vi "RampTestwithPlateau.vi"() -> ()   [LabVIEW 2016]
panel:
  in  "Plateau time (ms)":dbl=1.0
  out "Step seperation (us)":dbl=8.0
  in  "Ramp duration (us)":dbl=400.0 format="%#_6f"
  in  "Ramp trigger source":T1(ring)=enum."BNC_IN_A_RISING"
  in  "Step Size (Hz)":dbl=10000.0 format="%#_6f"
  in  "End Frequency (Hz)":dbl=700000.0 format="%#_13g"
  in  "Starting Frequency (Hz)":dbl=200000.0 format="%#_6f"
  in  "Channels":T2(ring)=enum."Channel 1"
  out "return count":u32=368
  out "error out":errorcluster={"status"=TRUE, "code"=-1073807339, "source"="VISA Read in RampTest.vi"}
  out "read buffer":string="DDS reset OK (0, 0)\r\n"
  out "Final instruction string":string="dds 1 reset\rdcp 1 spi:CFR2=0x1000080\rdcp 1 spi:STP0=0xD1B71\rdcp 1 wait:0h:\rdcp 1 update:u\rdcp 1 spi:DRL=0x2DE00D000D1B71\rdcp 1 spi:DRSS=0xA7C60000A7C6\rdcp 1 spi:DRR=0x7D007D0\rdcp 1 spi:CFR2=0x80080\rdcp 1 wait::BNC_IN_A_RISING\rdcp 1 update:u+d\rdcp 1 wait:50000h:\rdcp 1 update:u\rdcp 1 spi:CFR2=0x1000080\rdcp 1 spi:STP0=0x2DE00D\rdcp 1 wait:0h:\rdcp 1 update:u\rdcp 1 start\r"
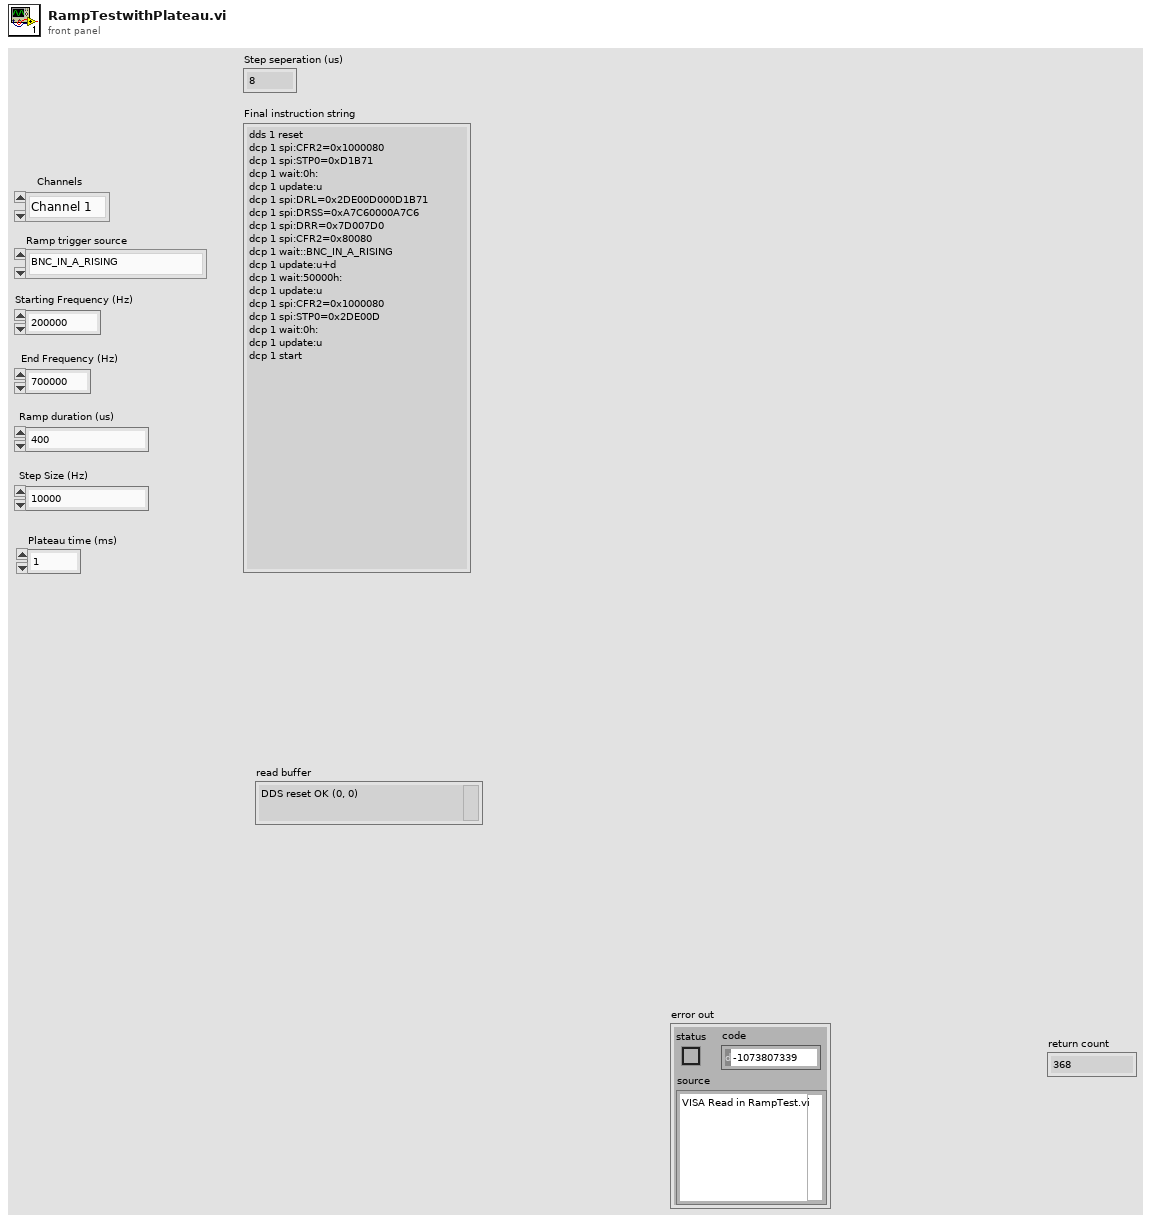
[diagram p1: front panel]
types:
  T1 = enum32{"O_RAMP_SWP_OVR", "RAM_SWP_OVR", "O_DROVER", "DROVER", "O_SPI_FIFO_EV1", "SPI_FIFO_EV1", "O_SPI_FIFO_EV0", "SPI_FIFO_EV0", "O_SPI_FIFO_FLUSHED", "SPI_FIFO_FLUSHED", "BNC_IN_B_LEVEL", "BNC_IN_B_FALLING", "BNC_IN_B_RISING", "BNC_IN_A_LEVEL", "BNC_IN_A_FALLING", "BNC_IN_A_RISING", "ALL_SPI_FIFOS_FLUSHED", "NONE"}
  T2 = enum32{"Channel 0", "Channel 1", "Both channels"}
  T3 = cluster{"Enable ASF from STP (F)":bool, "Digital ramp enable (F)":bool, "Digital ramp no-dwell high (F)":bool, "Digital ramp no-dwell low (F)":bool, "Matched latency enable (T)":bool, "Parallel data port enable (F)":bool}
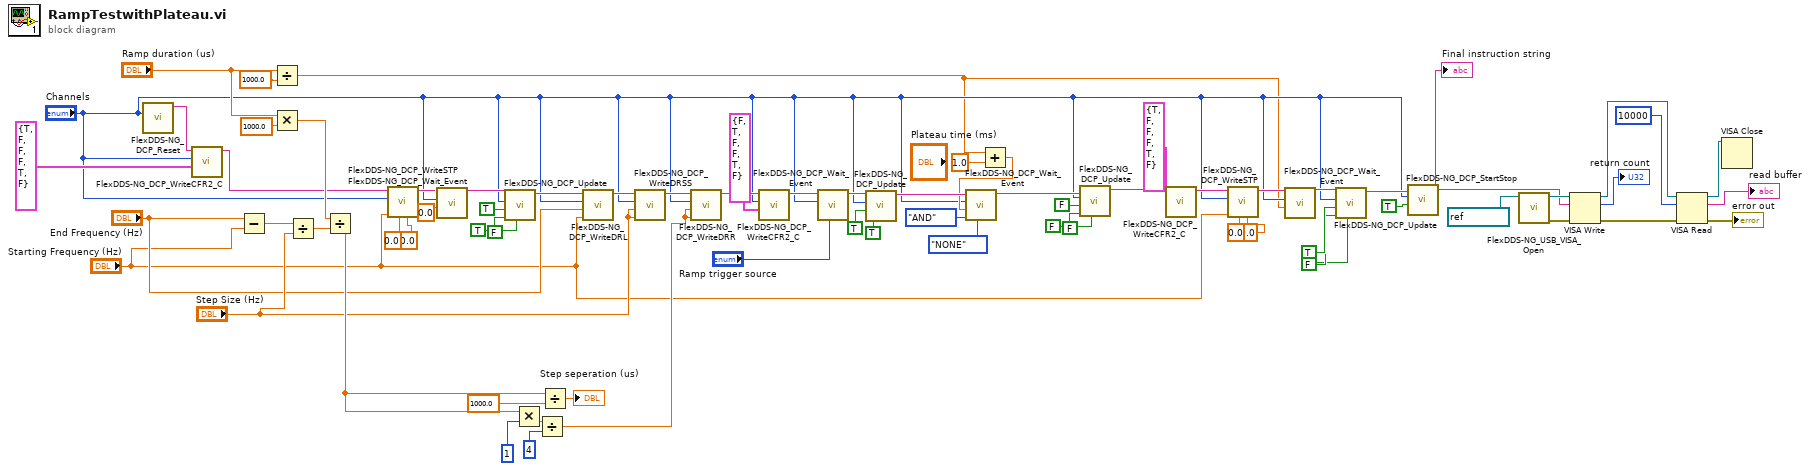
[diagram p0: block diagram]
diagram:
  n1 = call "FlexDDS-NG_DCP_Reset.vi"("Channels"="Channels") -> ("appended instruction string"=w22:string)  [unwired: 10 in]
  n2 = call "FlexDDS-NG_DCP_WriteCFR2_C.vi"("CFR2 bits"=T3 {"Enable ASF from STP (F)"=TRUE, "Digital ramp enable (F)"=FALSE, "Digital ramp no-dwell high (F)"=FALSE, "Digital ramp no-dwell low (F)"=FALSE, "Matched latency enable (T)"=TRUE, "Parallel data port enable (F)"=FALSE} ("CFR2 bits 2"), "Channels"="Channels", "initial instruction string"=w22) -> ("appended instruction string"=w23:string)  [unwired: 8 in]
  n3 = Subtract(x="End Frequency (Hz)", y="Starting Frequency (Hz)") -> (x-y=w35:dbl)
  n4 = Divide(x="Ramp duration (us)", y=1000.0) -> (x/y=w1:dbl)
  n5 = Multiply(x="Ramp duration (us)", y=1000.0) -> (x*y=w32:dbl)
  n6 = Divide(x=w35, y="Step Size (Hz)") -> (x/y=w33:dbl)
  n7 = Divide(x=w32, y=w33) -> (x/y=w31:dbl)
  n8 = call "FlexDDS-NG_DCP_WriteSTP.vi"("phase degrees (0..360)"=0.0, "amplitude (0..1)"=0.0, "frequency Hz (0..400M)"="Starting Frequency (Hz)", "Channels"="Channels", "initial instruction string"=w23) -> ("appended instruction string"=w16:string)  [unwired: 6 in]
  n9 = call "FlexDDS-NG_DCP_Wait_Event.vi"("waiting time [ms]"=0.0, "Channels in"="Channels", "appended instruction string in"=w16) -> ("appended instruction string"=w17:string)  [unwired: 8 in]
  n10 = call "FlexDDS-NG_DCP_Update.vi"("ONLY IO_UPDATE"=TRUE, "DRCTL(true=+, false=-)"=FALSE ("DRCTL(true=+, false=-) 2"), "IO_UPDATE(true=u, false = '')"=TRUE ("IO_UPDATE(true=u, false = '')  2"), "Channels"="Channels", "appended instruction string in"=w17) -> ("appended instruction string out"=w15:string)  [unwired: 6 in]
  n11 = Multiply(x=w31, y=u16 1) -> (x*y=w37:dbl)
  n12 = Divide(x=w37, y=u16 4) -> (x/y=w9:dbl)
  n13 = Divide(x=w31, y=1000.0 ("x/y")) -> (x/y=→"Step seperation (us)":dbl)
  n14 = call "FlexDDS-NG_DCP_WriteDRL.vi"("low limit"="Starting Frequency (Hz)", "high limit"="End Frequency (Hz)", "Channels"="Channels", "initial instruction string"=w15) -> ("appended instruction string"=w61:string)  [unwired: 7 in]
  n15 = call "FlexDDS-NG_DCP_WriteDRSS.vi"("increment step size"="Step Size (Hz)", "decrement step size"="Step Size (Hz)", "Channels"="Channels", "initial instruction string"=w61) -> ("appended instruction string"=w60:string)  [unwired: 7 in]
  n16 = call "FlexDDS-NG_DCP_WriteDRR.vi"("digital ramp positive slope rate"=w9, "digital ramp negative slope rate"=w9, "Channels"="Channels", "initial instruction string"=w60) -> ("appended instruction string"=w59:string)  [unwired: 7 in]
  n17 = call "FlexDDS-NG_DCP_WriteCFR2_C.vi"("CFR2 bits"=T3 {"Enable ASF from STP (F)"=FALSE, "Digital ramp enable (F)"=TRUE, "Digital ramp no-dwell high (F)"=FALSE, "Digital ramp no-dwell low (F)"=FALSE, "Matched latency enable (T)"=TRUE, "Parallel data port enable (F)"=FALSE}, "Channels"="Channels", "initial instruction string"=w59) -> ("appended instruction string"=w54:string)  [unwired: 8 in]
  n18 = call "FlexDDS-NG_DCP_Wait_Event.vi"("Event 1"="Ramp trigger source", "Channels in"="Channels", "appended instruction string in"=w54) -> ("appended instruction string"=w53:string)  [unwired: 8 in]
  n19 = call "FlexDDS-NG_DCP_Update.vi"("DRCTL(true=+, false=-)"=TRUE, "IO_UPDATE(true=u, false = '')"=TRUE, "Channels"="Channels", "appended instruction string in"=w53) -> ("appended instruction string out"=w48:string)  [unwired: 7 in]
  n20 = Add(x=w1, y=1.0) -> (x+y=w5:dbl)
  n21 = call "FlexDDS-NG_DCP_Wait_Event.vi"("Event 1"=T1."NONE", "AND/OR"=enum32{"AND", "OR"}."AND", "waiting time [ms]"=w5, "Channels in"="Channels", "appended instruction string in"=w48) -> ("appended instruction string"=w4:string)  [unwired: 6 in]
  n22 = call "FlexDDS-NG_DCP_Update.vi"("ONLY IO_UPDATE"=FALSE, "DRCTL(true=+, false=-)"=FALSE ("DRCTL(true=+, false=-) 2"), "IO_UPDATE(true=u, false = '')"=FALSE ("IO_UPDATE(true=u, false = '')  2"), "Channels"="Channels", "appended instruction string in"=w4) -> ("appended instruction string out"=w7:string)  [unwired: 6 in]
  n23 = call "FlexDDS-NG_DCP_WriteCFR2_C.vi"("CFR2 bits"=T3 {"Enable ASF from STP (F)"=TRUE, "Digital ramp enable (F)"=FALSE, "Digital ramp no-dwell high (F)"=FALSE, "Digital ramp no-dwell low (F)"=FALSE, "Matched latency enable (T)"=TRUE, "Parallel data port enable (F)"=FALSE}, "initial instruction string"=w7) -> ("appended instruction string"=w41:string)  [unwired: 9 in]
  n24 = call "FlexDDS-NG_DCP_WriteSTP.vi"("phase degrees (0..360)"=0.0, "amplitude (0..1)"=0.0, "frequency Hz (0..400M)"="Starting Frequency (Hz)", "Channels"="Channels", "initial instruction string"=w41) -> ("appended instruction string"=w40:string)  [unwired: 6 in]
  n25 = call "FlexDDS-NG_DCP_Wait_Event.vi"("waiting time [ms]"=w1, "Channels in"="Channels", "appended instruction string in"=w40) -> ("appended instruction string"=w39:string)  [unwired: 8 in]
  n26 = call "FlexDDS-NG_DCP_Update.vi"("ONLY IO_UPDATE"=TRUE, "DRCTL(true=+, false=-)"=FALSE ("DRCTL(true=+, false=-) 2"), "IO_UPDATE(true=u, false = '')"=TRUE ("IO_UPDATE(true=u, false = '')  2"), "Channels"="Channels", "appended instruction string in"=w39) -> ("appended instruction string out"=w44:string)  [unwired: 6 in]
  n27 = call "FlexDDS-NG_DCP_StartStop.vi"("start (T) stop (F)"=TRUE, "Channels"="Channels", "initial instruction string"=w44) -> ("appended instruction string"=w14:string)  [unwired: 8 in]
  "Final instruction string" <- w14
  n28 = call "FlexDDS-NG_USB_VISA_Open.vi"("FlexDDS-NG USB VISA resource name (COM)"=refnum<visa-resource-name> "COM7") -> ("error out"=w63:errorcluster, "FlexDDS-NG USB VISA resource name out"=w64:refnum<visa-resource-name>)  [unwired: 9 in]
  n29 = VISA Write(VISA resource name=w64, write buffer=w14, error in (no error)=w63) -> (VISA resource name out=w68:refnum<visa-resource-name>, return count=→"return count":u32, error out=w66:errorcluster)
  n30 = VISA Read(VISA resource name=w68, byte count=u32 10000, error in (no error)=w66) -> (VISA resource name out=w71:refnum<visa-resource-name>, read buffer=→"read buffer":string, error out=→"error out":errorcluster)  [unwired: 1 out]
  n31 = VISA Close(VISA resource name=w71) -> ()  [unwired: 1 in, 1 out]
